vi "FlushSink.vi"(8 "error in (no error)":errorcluster, 11 "Appender in":refnum<class "Appender.lvclass">) -> (0 "error out":errorcluster, 3 "Appender out":refnum<class "Appender.lvclass">)   [LabVIEW 2026, in "Lumberjack.lvlib" / "Appender.lvclass"]
doc: "Commit any buffered sink data to durable storage before the shutdown flush ack (flush fence, SRS-LMBR-002). Base is a no-op; only sinks with a write buffer override. Dynamic dispatch, protected."
uses:
  Appender.lvclass
  Appender.lvclass/Appender.ctl
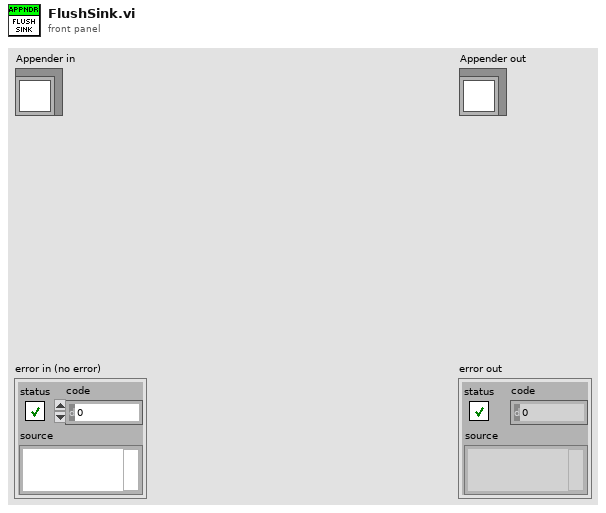
[diagram p1: front panel]
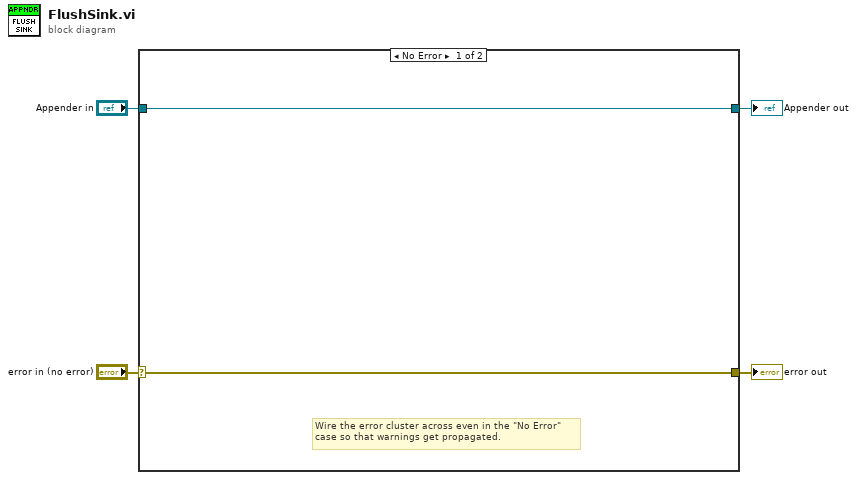
[diagram p0: block diagram]
diagram:
  n1 = case shown="No Error" "error in (no error)" {
    selector: "error in (no error)" -> [w5 w8]
    tunnel: [w5 w8] -> w3
    tunnel: [w6 w7] -> w1
    tunnel: "Appender in" -> [w6 w7]
    frame No Error {
      # "Wire the error cluster across even in the \"No Error\"\ncase so that warnings get propagated."
    }
    frame Error {
    }
  }
  "error out" <- w3
  "Appender out" <- w1
